vi "舵机手动 (子VI).vi"(0 "初始化":dbl, 1 "下限":dbl=0.1, 3 "上限":dbl=0.1, 5 "方向":bool[](array[boolean])=[FALSE, FALSE], 7 "加速率":dbl=100.0 format="%#_13g") -> (4 "PWM输出":dbl)   [LabVIEW 2017, in "年前程序.lvlib"]
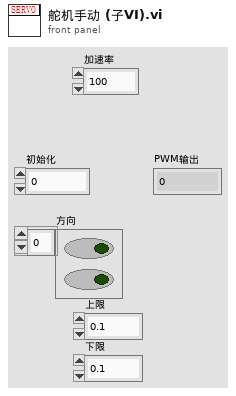
[diagram p1: front panel]
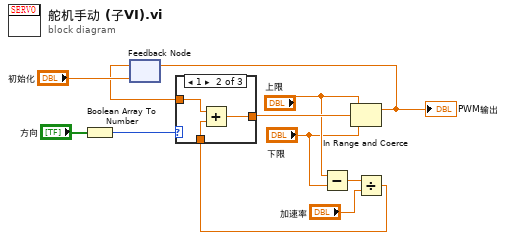
[diagram p0: block diagram]
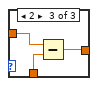
[diagram p3: hidden frame]
diagram:
  n1 = Boolean Array To Number(Boolean array="方向") -> (number=w9:u32)
  n2 = feedback #1("初始化") -> (w2:dbl)
  n3 = Subtract(x="上限", y="下限") -> (x-y=w4:dbl)
  n4 = Divide(x=w4, y="加速率") -> (x/y=w1:dbl)
  n5 = case shown="1" w9 {
    tunnel: [w12 w15 w17] -> w8
    tunnel: w2 -> [w12 w14 w18]
    tunnel: w1 -> [_ w13 w16]
    frame 0, Default {
    }
    frame 1 {
      n6 = Add(x=w14, y=w13) -> (x+y=w15:dbl)
    }
    frame 2 {
      n7 = Subtract(x=w18, y=w16) -> (x-y=w17:dbl)
    }
  }
  n8 = In Range and Coerce(upper limit="上限", x=w8, lower limit="下限") -> (coerced(x)=w7:dbl)  [unwired: 1 out]
  "PWM输出" <- w7
  n9 = feedback-in #1(w7) -> ()
